vi "niDTS WLAN OFDM Tx Test Get Default Limits.vi"(0 "Dummy Test Handle in":T13, 11 "error in (no error)":errorcluster) -> (4 "Dummy Test Handle out":T13, 6 "USL":T1 {"OBW"."Stop Frequency (Hz)" format="%#_4p"; "OBW"."Start Frequency (Hz)" format="%#_4p"; "OBW"."OBW (Hz)" format="%#_4p"}, 8 "LSL":T1 {"OBW"."Stop Frequency (Hz)" format="%#_4p"; "OBW"."Start Frequency (Hz)" format="%#_4p"; "OBW"."OBW (Hz)" format="%#_4p"}, 15 "error out":errorcluster)   [LabVIEW 2014, in "niDTS WLAN.lvlib"]
uses:
  niDTS WLAN.lvlib
  Tx Test/Includes/niDTS WLAN Tx Test INC Handle.ctl
  Tx Test/Objects/BASE_class/niDTS WLAN Tx Test.lvclass
  Tx Test/Includes/niDTS WLAN Tx Test INC Results.ctl
  Tx Test/Includes/niDTS WLAN Tx Test INC MOD EVM Results.ctl
  Tx Test/Includes/Results/niDTS Tx RES INC EVM.ctl
  Tx Test/Includes/niDTS WLAN Tx Test INC TXP Results.ctl
  Tx Test/Includes/niDTS WLAN Tx Test INC TXP Result SINGLE.ctl
  Tx Test/Includes/niDTS WLAN Tx Test INC OBW Results.ctl
  Instrument/INSTR TX/Results/niDTS WLAN INSTR TX INC SEM Results.ctl
  Instrument/INSTR TX/Results/niDTS WLAN INSTR TX INC SEM FSEGemts Results.ctl
  Tx Test/Includes/Results/niDTS Tx RES INC SEM FSEGemts.ctl
  Instrument/INSTR TX/Results/niDTS WLAN INSTR TX INC SEM MARGin Results.ctl
  Tx Test/Includes/Results/niDTS Tx RES INC SEM Margin.ctl
  Instrument/INSTR TX/Results/niDTS WLAN INSTR TX INC OFDM Impairments Results.ctl
  Instrument/INSTR TX/niDTS WLAN INSTR TX.lvclass
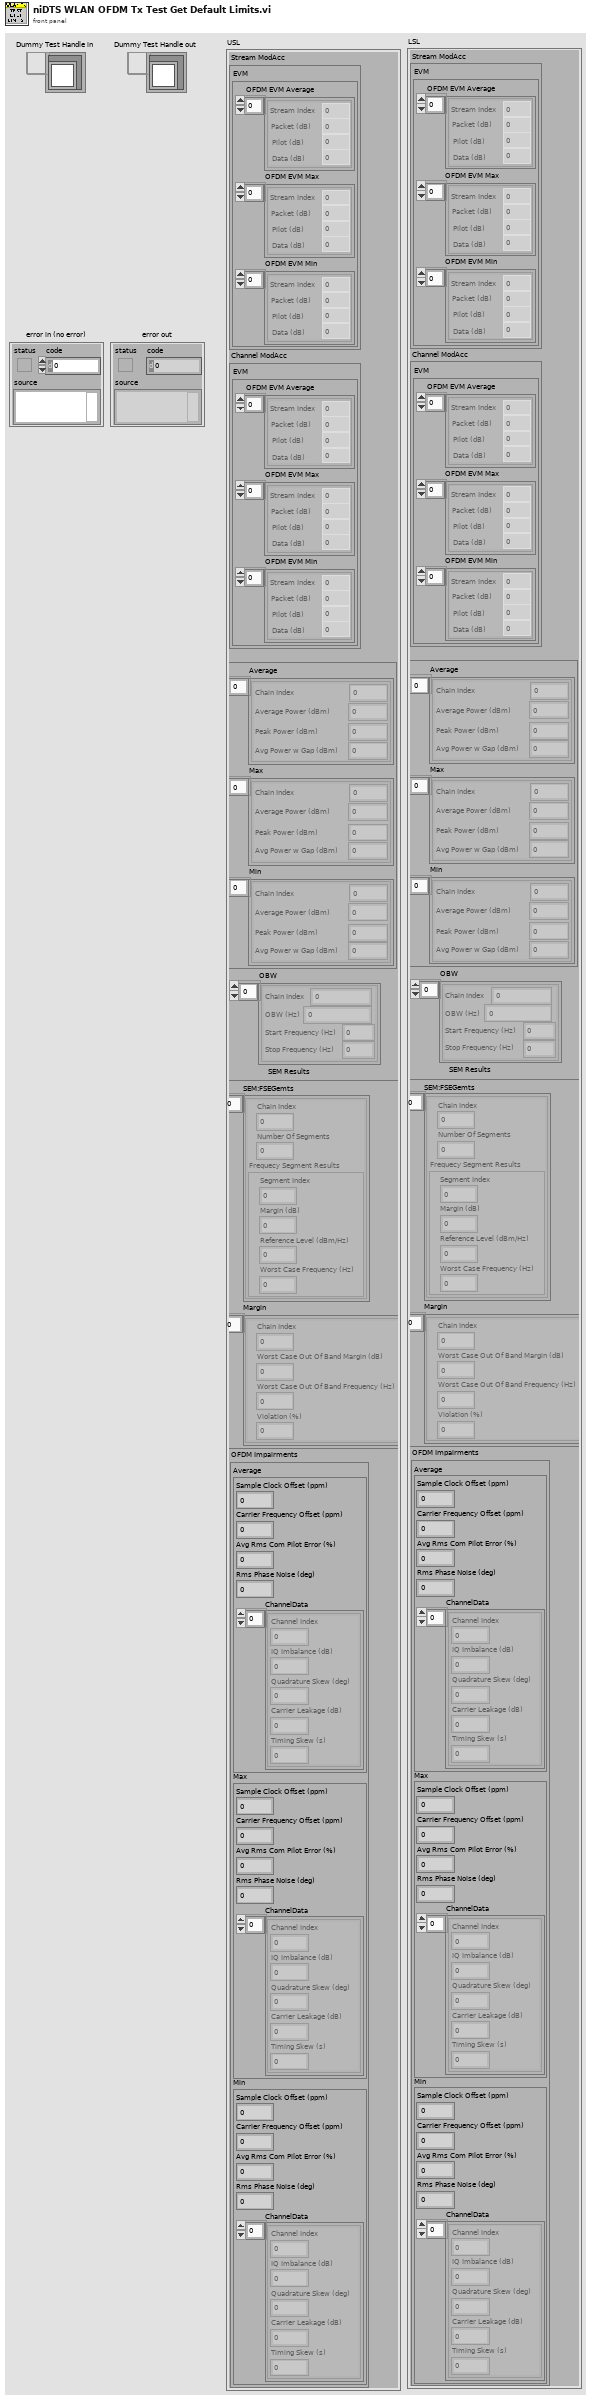
[diagram p1: front panel]
types:
  T1 = typedef "niDTS WLAN.lvlib/niDTS WLAN Tx Test INC Results.ctl" = cluster{"Stream ModAcc":T2, "Channel ModAcc":T2, "TXP":T4, "OBW":T6[], "SEM Results":T7, "OFDM Impairments":T12}
  T2 = typedef "niDTS WLAN.lvlib/niDTS WLAN Tx Test INC MOD EVM Results.ctl" = cluster{"EVM":cluster{"OFDM EVM Average":T3[], "OFDM EVM Max":T3[], "OFDM EVM Min":T3[]}}
  T3 = typedef "niDTS WLAN.lvlib/niDTS Tx RES INC EVM.ctl" = cluster{"Stream Index":i32, "Packet (dB)":dbl, "Pilot (dB)":dbl, "Data (dB)":dbl}
  T4 = typedef "niDTS WLAN.lvlib/niDTS WLAN Tx Test INC TXP Results.ctl" = cluster{"Average":T5[], "Max":T5[], "Min":T5[]}
  T5 = typedef "niDTS WLAN.lvlib/niDTS WLAN Tx Test INC TXP Result SINGLE.ctl" = cluster{"Chain Index":dbl, "Average Power (dBm)":dbl, "Peak Power (dBm)":dbl, "Avg Power w Gap (dBm)":dbl}
  T6 = typedef "niDTS WLAN.lvlib/niDTS WLAN Tx Test INC OBW Results.ctl" = cluster{"Chain Index":dbl, "OBW (Hz)":dbl, "Start Frequency (Hz)":dbl, "Stop Frequency (Hz)":dbl}
  T7 = typedef "niDTS WLAN.lvlib/niDTS WLAN INSTR TX.lvclass/niDTS WLAN INSTR TX INC SEM Results.ctl" = cluster{"SEM:FSEGemts":T8, "Margin":T10}
  T8 = typedef "niDTS WLAN.lvlib/niDTS WLAN INSTR TX.lvclass/niDTS WLAN INSTR TX INC SEM FSEGemts Results.ctl" = T9[]
  T9 = typedef "niDTS WLAN.lvlib/niDTS Tx RES INC SEM FSEGemts.ctl" = cluster{"Chain Index":i32, "Number Of Segments":i32, "Frequecy Segment Results":cluster{"Segment Index":i32, "Margin (dB)":dbl, "Reference Level (dBm/Hz)":dbl, "Worst Case Frequency (Hz)":dbl}}
  T10 = typedef "niDTS WLAN.lvlib/niDTS WLAN INSTR TX.lvclass/niDTS WLAN INSTR TX INC SEM MARGin Results.ctl" = T11[]
  T11 = typedef "niDTS WLAN.lvlib/niDTS Tx RES INC SEM Margin.ctl" = cluster{"Chain Index":i32, "Worst Case Out Of Band Margin (dB)":dbl, "Worst Case Out Of Band Frequency (Hz)":dbl, "Violation (%)":dbl}
  T12 = typedef "niDTS WLAN.lvlib/niDTS WLAN INSTR TX.lvclass/niDTS WLAN INSTR TX INC OFDM Impairments Results.ctl" = cluster{"Average":cluster{"Sample Clock Offset (ppm)":dbl, "Carrier Frequency Offset (ppm)":dbl, "Avg Rms Com Pilot Error (%)":dbl, "Rms Phase Noise (deg)":dbl, "ChannelData":cluster{"Channel Index":i32, "IQ Imbalance (dB)":dbl, "Quadrature Skew (deg)":dbl, "Carrier Leakage (dB)":dbl, "Timing Skew (s)":dbl}[]}, "Max":cluster{"Sample Clock Offset (ppm)":dbl, "Carrier Frequency Offset (ppm)":dbl, "Avg Rms Com Pilot Error (%)":dbl, "Rms Phase Noise (deg)":dbl, "ChannelData":cluster{"Channel Index":i32, "IQ Imbalance (dB)":dbl, "Quadrature Skew (deg)":dbl, "Carrier Leakage (dB)":dbl, "Timing Skew (s)":dbl}[]}, "Min":cluster{"Sample Clock Offset (ppm)":dbl, "Carrier Frequency Offset (ppm)":dbl, "Avg Rms Com Pilot Error (%)":dbl, "Rms Phase Noise (deg)":dbl, "ChannelData":cluster{"Channel Index":i32, "IQ Imbalance (dB)":dbl, "Quadrature Skew (deg)":dbl, "Carrier Leakage (dB)":dbl, "Timing Skew (s)":dbl}[]}}
  T13 = typedef "niDTS WLAN.lvlib/niDTS WLAN Tx Test INC Handle.ctl" = refnum<data-value>
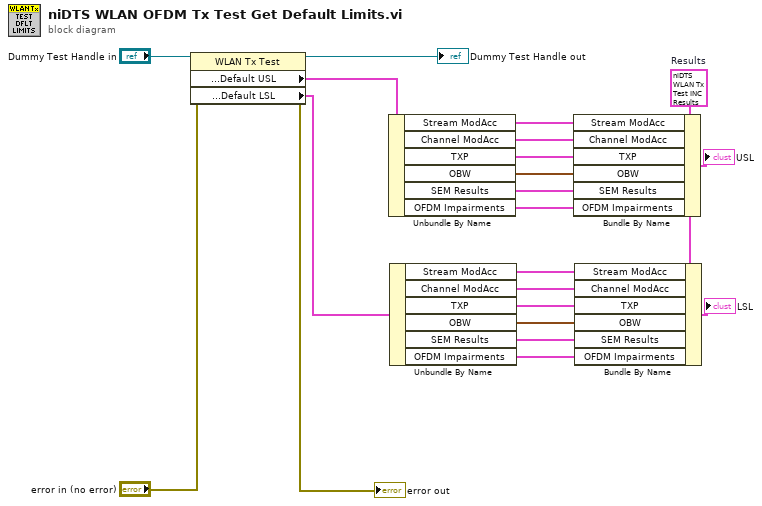
[diagram p0: block diagram]
diagram:
  w4 = T1 {"Stream ModAcc"={"EVM"={"OFDM EVM Average"=[], "OFDM EVM Max"=[], "OFDM EVM Min"=[]}}, "Channel ModAcc"={"EVM"={"OFDM EVM Average"=[], "OFDM EVM Max"=[], "OFDM EVM Min"=[]}}, "TXP"={"Average"=[], "Max"=[], "Min"=[]}, "OBW"=[], "SEM Results"={"SEM:FSEGemts"=[], "Margin"=[]}, "OFDM Impairments"={"Average"={"Sample Clock Offset (ppm)"=0.0, "Carrier Frequency Offset (ppm)"=0.0, "Avg Rms Com Pilot Error (%)"=0.0, "Rms Phase Noise (deg)"=0.0, "ChannelData"=[]}, "Max"={"Sample Clock Offset (ppm)"=0.0, "Carrier Frequency Offset (ppm)"=0.0, "Avg Rms Com Pilot Error (%)"=0.0, "Rms Phase Noise (deg)"=0.0, "ChannelData"=[]}, "Min"={"Sample Clock Offset (ppm)"=0.0, "Carrier Frequency Offset (ppm)"=0.0, "Avg Rms Com Pilot Error (%)"=0.0, "Rms Phase Noise (deg)"=0.0, "ChannelData"=[]}}}  # Results
  n1 = property class="WLAN Tx Test"(reference="Dummy Test Handle in", error in="error in (no error)") -> (reference out=→"Dummy Test Handle out":T13, error out=→"error out":errorcluster, "Properties:Default Limits:Default USL"=w17:T1, "Properties:Default Limits:Default LSL"=w6:T1)
  n2 = Unbundle By Name(w17) -> ("Stream ModAcc"=w13:T2, "Channel ModAcc"=w12:T2, "TXP"=w14:T4, "OBW"=w15:T6[], "SEM Results"=w16:T7, "OFDM Impairments"=w2:T12)
  n3 = Unbundle By Name(w6) -> ("Stream ModAcc"=w10:T2, "Channel ModAcc"=w11:T2, "TXP"=w9:T4, "OBW"=w8:T6[], "SEM Results"=w7:T7, "OFDM Impairments"=w1:T12)
  n4 = Bundle By Name(cluster=w4, "Stream ModAcc"=w13, "Channel ModAcc"=w12, "TXP"=w14, "OBW"=w15, "SEM Results"=w16, "OFDM Impairments"=w2) -> (→"USL":T1)
  n5 = Bundle By Name(cluster=w4, "Stream ModAcc"=w10, "Channel ModAcc"=w11, "TXP"=w9, "OBW"=w8, "SEM Results"=w7, "OFDM Impairments"=w1) -> (→"LSL":T1)
